vi "STM Write Meta Data (UDP Ref).vi"(4 "Address":cluster{"address":u32, "port":u16}, 6 "Options":T1={"Ignore Timeout Error"=TRUE, "timeout ms (1000)"=1000}, 7 "Meta data":T3[](array[typedef]), 8 "error in":errorcluster, 11 "connection ID":refnum<k16>) -> (0 "error out":errorcluster, 3 "Connection Info Out":T2)   [LabVIEW 2014, in "QwaveSys Raspberry Pi Library.lvlib"]
doc: "Use this VI to transmit the meta data cluster to a remote computer. Sending the meta data to another computer helps maintainability since the data resides only on one side and it is shared to other computers at run time."
uses:
  QwaveSys Raspberry Pi Library.lvlib
  _SubVIs/stm_MetaDataElement.ctl
  stm_UDP Connection Info.ctl
  stm_UDP Write Options.ctl
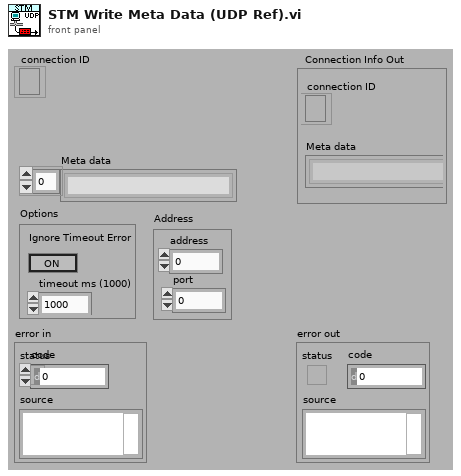
[diagram p1: front panel]
types:
  T1 = typedef "QwaveSys Raspberry Pi Library.lvlib/stm_UDP Write Options.ctl" = cluster{"Ignore Timeout Error":bool, "timeout ms (1000)":i32}
  T2 = typedef "QwaveSys Raspberry Pi Library.lvlib/stm_UDP Connection Info.ctl" = cluster{"connection ID":refnum<k16>, "Meta data":T3[]}
  T3 = typedef "QwaveSys Raspberry Pi Library.lvlib/stm_MetaDataElement.ctl" = string
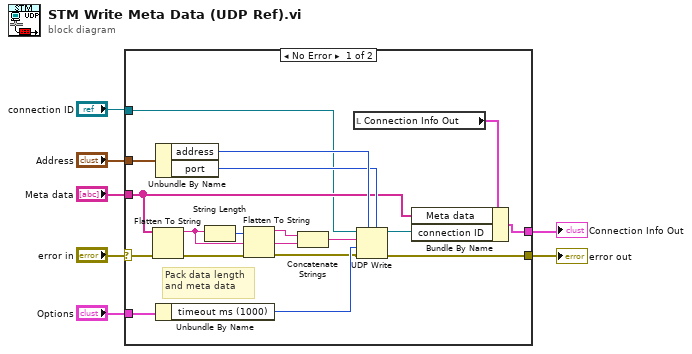
[diagram p0: block diagram]
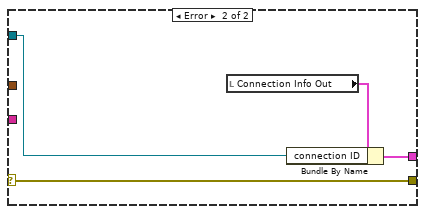
[diagram p2: hidden frame]
diagram:
  n1 = case shown="No Error" "error in" {
    selector: "error in" -> [w13 w29]
    tunnel: [w14 w26] -> w7
    tunnel: "connection ID" -> [w9 w27]
    tunnel: "Meta data" -> [w10 _]
    tunnel: [w22 w29] -> w5
    tunnel: "Address" -> [w20 _]
    tunnel: "Options" -> [w17 _]
    frame No Error {
      # "Pack data length\nand meta data"
      n2 = Flatten To String(anything=w10, error in (no error)=w13) -> (data string=w23:string, error out=w12:errorcluster)  [unwired: 3 out]
      n3 = Unbundle By Name(w20) -> ("address"=w19:u32, "port"=w18:u16)
      n4 = Unbundle By Name(w17) -> ("timeout ms (1000)"=w16:i32)
      n5 = String Length(string=w23) -> (length=w25:i32)
      n6 = Flatten To String(anything=w25, error in (no error)=w12) -> (data string=w24:string, error out=w11:errorcluster)  [unwired: 3 out]
      n7 = Concatenate Strings(w24, w23) -> (w21:string)
      n8 = local read "Connection Info Out"() -> (w8:T2)
      n9 = UDP Write(address=w19, port or service name=w18, connection ID=w9, data in=w21, 8:w11, 9:w16) -> (error out=w22:errorcluster, 3:w15:refnum<k16>)
      n10 = Bundle By Name(cluster=w8, "Meta data"=w10, "connection ID"=w15) -> (w14:T2)
    }
    frame Error {
      n11 = local read "Connection Info Out"() -> (w28:T2)
      n12 = Bundle By Name(cluster=w28, "connection ID"=w27) -> (w26:T2)
    }
  }
  "error out" <- w5
  "Connection Info Out" <- w7
